vi "Set Command Error.vi"(4 "Source (\"\")":string, 8 "error in (no error)":errorcluster, 11 "VISA resource name":refnum<visa-resource-name>) -> (0 "error out":errorcluster, 3 "VISA resource name out":refnum<visa-resource-name>)   [LabVIEW 2011, in "Yokogawa DX Series.lvlib"]
doc: "This VI sets an error.\n\"command are not processed succesfully\"."
uses:
  <instrlib>/Yokogawa DX Series/Yokogawa DX Series.lvlib
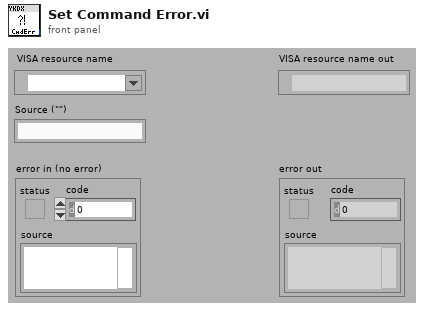
[diagram p1: front panel]
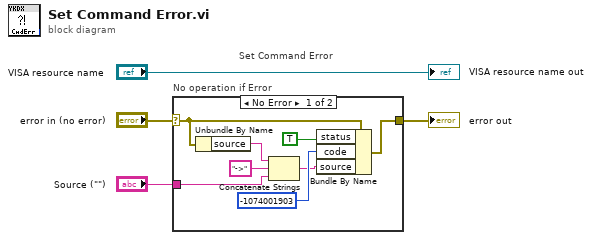
[diagram p0: block diagram]
diagram:
  # "Set Command Error"
  n1 = case "No operation if Error" shown="No Error" "error in (no error)" {
    selector: "error in (no error)" -> [w9 w13]
    tunnel: [w12 w13] -> w3
    tunnel: "Source (\"\")" -> [w6 _]
    frame No Error {
      n2 = Unbundle By Name(w9) -> ("source"=w8:string)
      n3 = Concatenate Strings(w8, "->", w6) -> (w5:string)
      n4 = Bundle By Name(cluster=w9, "status"=TRUE, "code"=-1074001903, "source"=w5) -> (w12:errorcluster)
    }
    frame Error {
    }
  }
  "error out" <- w3
  "VISA resource name out" <- "VISA resource name"
